vi "U6 Multiple AIN Example eAddGoGet.vi"() -> ()   [LabVIEW 2021]
panel:
  in  "Binary":bool
  in  "SettlingFactor":i32
  in  "Negative Channels":i32[](array[numeric])=[0, 0, 0, 0]
  in  "Ranges":string[](array[string])=["LJ_rgBIP10V", "LJ_rgBIP10V", "LJ_rgBIPP01V", "LJ_rgBIPP01V"]
  in  "Positive Channels":i32[](array[numeric])=[0, 1, 2, 3]
  out "Values Read":dbl[](array[numeric]) format="%.6f"
  out "Error Message":string
  in  "Resolution":i32
  out "error out":errorcluster
  # "Aquires multiple analog input channels over USB from the first found U6.\n\nThis uses eAddGoGet from the UD driver, rather than the LabVIEW utility AddS-Go-Get.vi.  The utility\nVI has better/easier error handling and is normally preferred, but eAddGoGet is a single call to the UD driver\nso often preferred if you will have parallel driver calls to the same handle within the same thread (none of\nour examples do this)."
  # "LJ_rgBIP10V\nLJ_rgBIP1V\nLJ_rgBIPP1V\nLJ_rgBIPP01V"
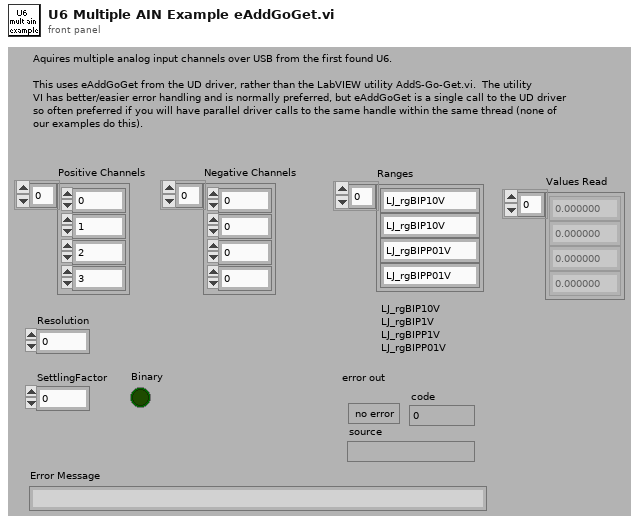
[diagram p1: front panel]
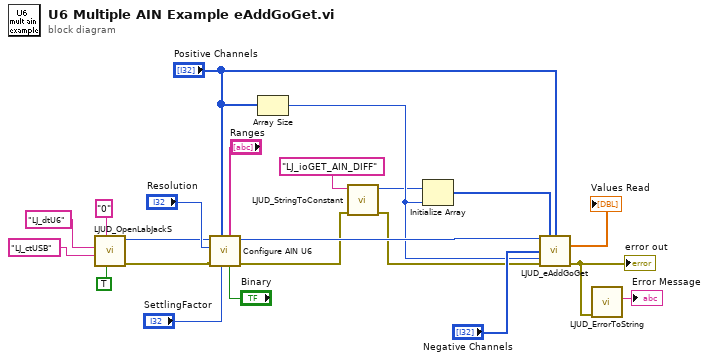
[diagram p0: block diagram]
diagram:
  n1 = call "LJUD_OpenLabJackS.vi"("FirstFound"=TRUE, "Address"="0", "ConnectionType"="LJ_ctUSB", "DeviceType"="LJ_dtU6") -> ("error out"=w11:errorcluster, "Handle"=w12:i32)  [unwired: 5 in, 1 out]
  n2 = call "Configure AIN U6.vi"("Binary"="Binary", "Ranges"="Ranges", "SettlingFactor"="SettlingFactor", "Positive Channels"="Positive Channels", "error in"=w11, "Resolution"="Resolution", "Handle In"=w12) -> ("error out"=w7:errorcluster, "Handle Out"=w20:i32)  [unwired: 3 in]
  n3 = Array Size(array="Positive Channels") -> (size(s)=w4:i32)
  n4 = call "LJUD_StringToConstant.vi"("error in"=w7, "String"="LJ_ioGET_AIN_DIFF" ("IOType")) -> ("error out"=w6:errorcluster, "Constant Number"=w3:i32)  [unwired: 8 in]
  n5 = Initialize Array(w3, w4) -> (w2:i32[])
  n6 = call "LJUD_eAddGoGet.vi"("Handle In"=w20, "aIOTypes"=w2, "aChannels"="Positive Channels", "ax1s"="Negative Channels", "NumRequests"=w4, "error in"=w6) -> ("Values Read"=→"Values Read":dbl[], "error out"=w19:errorcluster)  [unwired: 4 in, 4 out]
  "error out" <- w19
  n7 = call "LJUD_ErrorToString.vi"("error in"=w19) -> ("String"=→"Error Message":string)  [unwired: 10 in]
